vi "Projecte 1.2.vi"() -> ()   [LabVIEW 2014]
uses:
  <vilib>/LabVIEW Hacker/LINX/Public/Peripherals/PWM/Set Duty Cycle 1 Chan.vi
  <vilib>/LabVIEW Hacker/LINX/Public/Peripherals/Analog/Analog Read 1 Chan.vi
  <vilib>/LabVIEW Hacker/LINX/LVH-LINX.lvlib
panel:
  in  "stop":bool
  in  "Nombre corbes":i32=2
  out "XY Graph":cluster{dbl[], dbl[]}[](graph)
  out "error out":errorcluster
  in  "access (0:read/write)":enum16{"read/write", "read-only", "write-only"}(ring)
  in  "operation (0:open)":T1(ring)
  in  "file path (use dialog)":path
  out "Error Out":errorcluster
  in  "Serial Port":refnum<visa-resource-name>="N/A"
  out "duty cycle":dbl
  in  "Mesures":i32
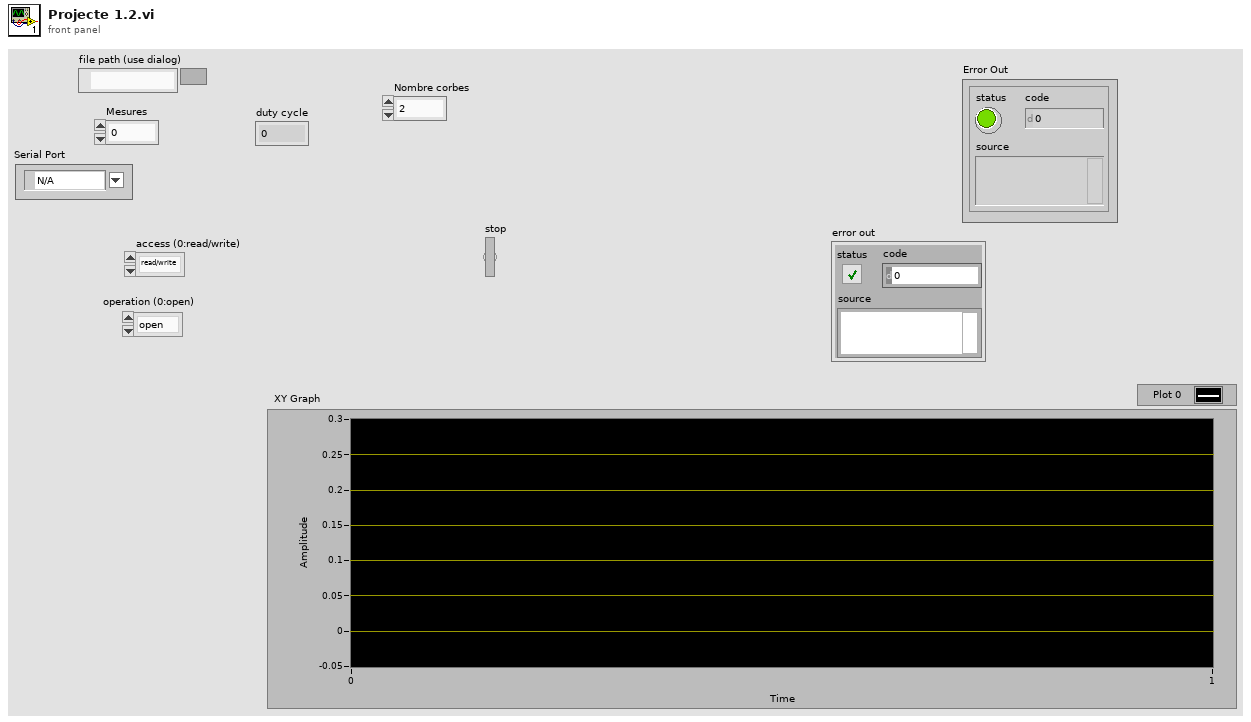
[diagram p1: front panel]
types:
  T1 = enum16{"open", "replace", "create", "open or create", "replace or create", "replace or create with confirmation"}
  T2 = typedef "LVH-LINX.lvlib/LINX Ref.ctl" = cluster{"Platform":T3, "Interface":T4, "LINX Device Config":T5}
  T3 = typedef "LVH-LINX.lvlib/Platform.ctl" = enum16{"LINX", "myRIO"}
  T4 = typedef "LVH-LINX.lvlib/Interface.ctl" = enum16{"Serial", "TCP"}
  T5 = typedef "LVH-LINX.lvlib/Device.lvlib/LINX Device Config.ctl" = cluster{"Interface":T4, "COM Port":refnum<visa-resource-name>, "TCP Configuration":T6, "Device Family":T7, "Device ID":u8, "Device Name":string, "TCP Ref":refnum<k5>}
  T6 = typedef "LVH-LINX.lvlib/Device.lvlib/TCP Config.ctl" = cluster{"IP Address":string, "Port":u16}
  T7 = typedef "LVH-LINX.lvlib/Device Family.ctl" = enum8{"National Instruments", "Digilent", "Arduino"}
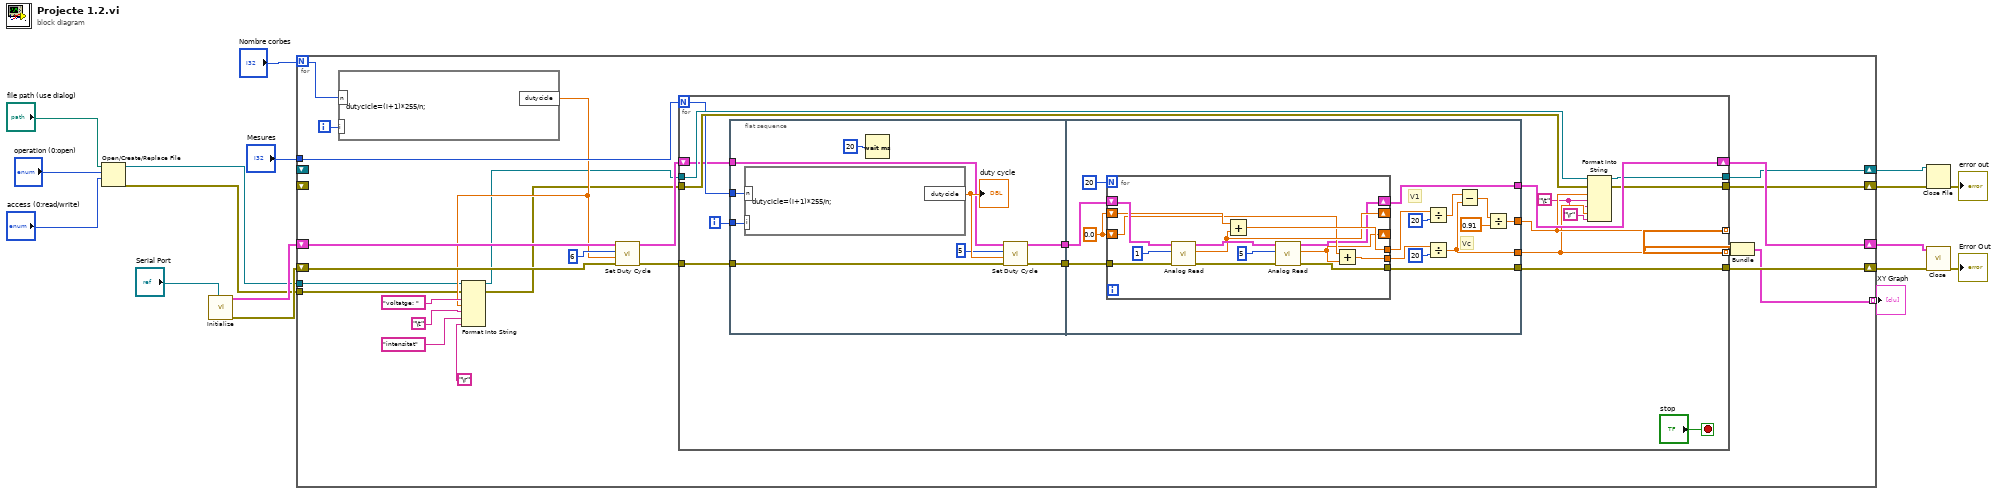
[diagram p0: block diagram]
diagram:
  n1 = Open/Create/Replace File(file path (use dialog)="file path (use dialog)", operation (0:open)="operation (0:open)", access (0:read/write)="access (0:read/write)") -> (refnum out=w2:refnum<file>, error out=w1:errorcluster)  [unwired: 3 in, 1 out]
  n2 = call <vilib>:"Initialize.vi"("Serial Port"="Serial Port") -> ("Error Out"=w13:errorcluster, "LINX Ref"=w17:T2)  [unwired: 8 in, 1 out]
  n3 = for {
    N: "Nombre corbes" -> [w29]
    tunnel: "Mesures" -> [w41]
    shift-right: [w40] -> w15
    shift-left: w17 -> [w34]
    shift-right: [w39] -> w12
    shift-left: w13 -> [w32]
    shift-right: [w38] -> w7
    shift-left: _ -> [_]
    shift-right: [w37] -> w6
    shift-left: _ -> [_]
    tunnel: [w36] -> w3 mode=indexing
    tunnel: w2 -> [w22]
    tunnel: w1 -> [w21]
    i -> [w30]
    n4 = formula code="dutycicle=(i+1)*255/n;"("i"=w30, "n"=w29) -> ("dutycicle"=w23:dbl)
    n5 = Format Into String(initial string=w22, error in=w21, "voltatge: " ("String"), w23, "\t", "intensitat" ("String"), "\r") -> (resulting string=w20:refnum<file>, error out=w19:errorcluster)  [unwired: 1 in]
    n6 = call-poly <vilib>:"Set Duty Cycle.vi"("Error In"=w32, "Duty Cycle"=w23, "PWM Channel"=u8 6, "LINX Resource"=w34) -> ("Error Out"=w31:errorcluster, "LINX Resource"=w33:T2)  [unwired: 6 in]
    n7 = for {
      N: w41 -> [w49]
      shift-right: [w57] -> w40
      shift-left: w33 -> [w48]
      tunnel: w31 -> [w47]
      tunnel: [w54] -> w39
      tunnel: w20 -> [w53]
      tunnel: w19 -> [w52]
      tunnel: [w51] -> w38
      tunnel: [w50] -> w37
      tunnel: [w46] -> w28 mode=indexing
      tunnel: [w44] -> w27 mode=indexing
      i -> [w56]
      stop <- "stop" stop-if-true
      w43 = "\t"
      n8 = flat-sequence {
        tunnel: [w66] -> w58
        tunnel: w56 -> [w61]
        tunnel: [w63] -> w55
        tunnel: w49 -> [w62]
        tunnel: w48 -> [w60]
        tunnel: w47 -> [w59]
        tunnel: w58 -> [w76]
        tunnel: [w75] -> w57
        tunnel: [w70] -> w44
        tunnel: [w68] -> w46
        tunnel: w55 -> [w72]
        tunnel: [w71] -> w54
        frame #0 {
          n9 = formula code="dutycicle=(i+1)*255/n;"("i"=w61, "n"=w62) -> ("dutycicle"=w65:dbl)
          "duty cycle" <- w65
          n10 = Wait (ms)(milliseconds to wait=u32 20) -> ()  [unwired: 1 out]
          n11 = call-poly <vilib>:"Set Duty Cycle.vi"("Error In"=w59, "Duty Cycle"=w65, "PWM Channel"=u8 5, "LINX Resource"=w60) -> ("Error Out"=w63:errorcluster, "LINX Resource"=w66:T2)  [unwired: 6 in]
        }
        frame #1 {
          w79 = 0.0
          # "Vc"
          # "V1"
          n12 = for {
            N: 20 -> [_]
            shift-right: [w87] -> w75
            shift-left: w76 -> [w96]
            shift-right: [w91] -> _
            shift-left: w79 -> [w93]
            tunnel: [w92] -> w81
            shift-right: [w89] -> _
            shift-left: w79 -> [w90]
            tunnel: [w88] -> w77
            tunnel: w72 -> [w86]
            tunnel: [w84] -> w71
            n13 = call-poly <vilib>:"Analog Read.vi"("Error In"=w86, "Analog Channel"=u8 1, "LINX Resource"=w96) -> ("Error Out"=w85:errorcluster, "AI Value"=w91:dbl, "LINX Resource"=w94:T2)  [unwired: 5 in, 1 out]
            n14 = Add(x=w93, y=w91) -> (x+y=w92:dbl)
            n15 = call-poly <vilib>:"Analog Read.vi"("Error In"=w85, "Analog Channel"=u8 5, "LINX Resource"=w94) -> ("Error Out"=w84:errorcluster, "AI Value"=w89:dbl, "LINX Resource"=w87:T2)  [unwired: 5 in, 1 out]
            n16 = Add(x=w90, y=w89) -> (x+y=w88:dbl)
          }
          n17 = Divide(x=w81, y=20) -> (x/y=w69:dbl)
          n18 = Divide(x=w77, y=20) -> (x/y=w70:dbl)
          n19 = Subtract(x=w69, y=w70) -> (x-y=w74:dbl)
          n20 = Divide(x=w74, y=0.91) -> (x/y=w68:dbl)
        }
      }
      n21 = Format Into String(initial string=w53, error in=w52, w46, w43, w43, w44, "\r") -> (resulting string=w51:refnum<file>, error out=w50:errorcluster)  [unwired: 1 in]
    }
    n22 = Bundle(w27, w28) -> (w36:cluster{dbl[], dbl[]})  [unwired: 1 in]
  }
  "XY Graph" <- w3
  n23 = Close File(refnum=w7, error in=w6) -> (error out=→"error out":errorcluster)  [unwired: 1 out]
  n24 = call <vilib>:"Close.vi"("Error In"=w12, "LINX Resource"=w15) -> ("Error Out"=→"Error Out":errorcluster)  [unwired: 8 in, 1 out]
